vi "Read Data Strings.vi"(8 "error in (no error)":errorcluster, 11 "Build Named Build Specification in":refnum<class "Build Named Build Specification.lvclass">) -> (0 "error out":errorcluster, 1 "Target Name":string, 2 "Build Specification Name":string, 3 "Build Named Build Specification out":refnum<class "Build Named Build Specification.lvclass">)   [LabVIEW 2020, in "ProjectBuilder.lvlib" / "Build Named Build Specification.lvclass"]
doc: "Read private data."
uses:
  Build Named Build Specification.lvclass
  Build Named Build Specification.lvclass/Build Named Build Specification.ctl
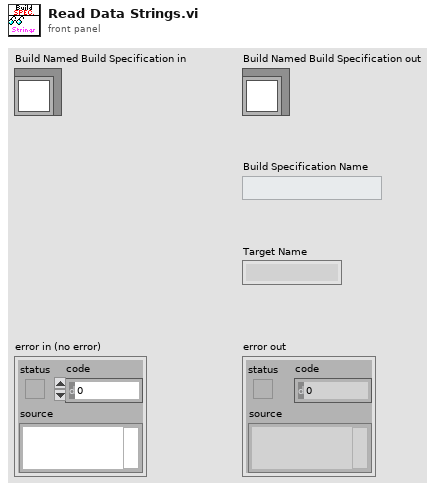
[diagram p1: front panel]
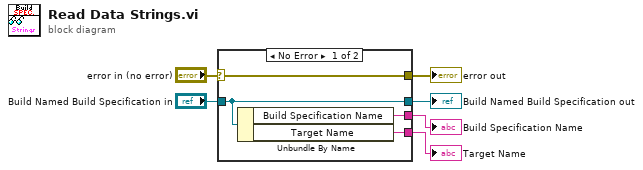
[diagram p0: block diagram]
diagram:
  n1 = case shown="No Error" "error in (no error)" {
    selector: "error in (no error)" -> [w10 w11]
    tunnel: [w10 w11] -> w5
    tunnel: [w9 w12] -> w3
    tunnel: "Build Named Build Specification in" -> [w9 w12]
    tunnel: [w8 _] -> w2
    tunnel: [w7 _] -> w1
    frame No Error {
      n2 = Unbundle By Name(w9) -> ("Build Specification Name"=w8:string, "Target Name"=w7:string)
    }
    frame Error {
    }
  }
  "error out" <- w5
  "Build Named Build Specification out" <- w3
  "Build Specification Name" <- w2
  "Target Name" <- w1
